vi "ChartExample.vi"() -> ()   [LabVIEW 2012]
panel:
  out "Waveform Chart":dbl(graph)
  in  "stop":bool
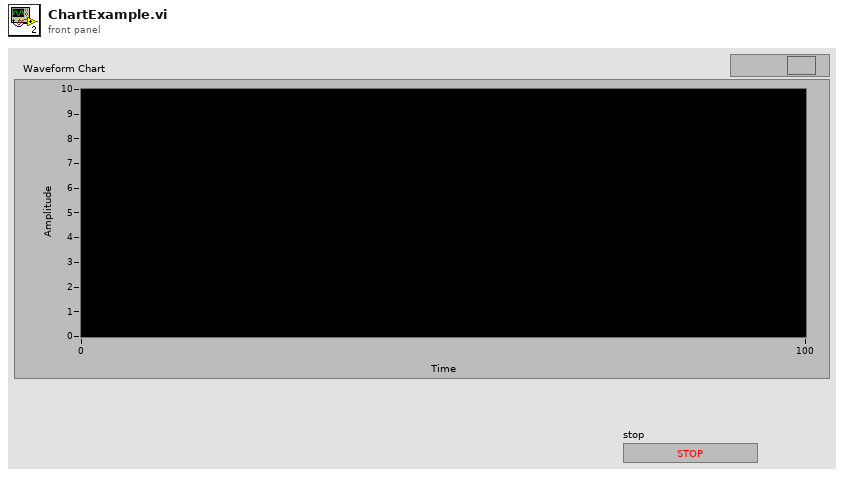
[diagram p1: front panel]
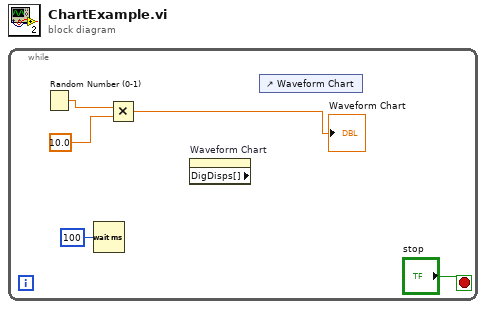
[diagram p0: block diagram]
diagram:
  n1 = while {
    stop <- "stop" stop-if-true
    n2 = Random Number (0-1)() -> (number: 0 to 1=w4:dbl)
    n3 = Wait (ms)(milliseconds to wait=u32 100) -> ()  [unwired: 1 out]
    n4 = Multiply(x=w4, y=10.0) -> (x*y=→"Waveform Chart":dbl)
    n5 = property on="Waveform Chart" class="WFChart (strict)" props=["DigDisps[]"]() -> ()  [unwired: 2 in, 3 out]
    n6 = control-ref of="Waveform Chart"() -> ()  [unwired: 1 out]
  }
